vi "Pre Launch Init.vi"(11 "仿真双风扇":refnum<class "Simulated Dual Fan.lvclass">) -> (0 "error out":cluster{"状态":bool, "代码":i32, "源":string} caption="错误输出", 3 "仿真双风扇":refnum<class "Simulated Dual Fan.lvclass">)   [LabVIEW 2015, in "Simulated Dual Fan.lvclass"]
uses:
  Simulated Dual Fan.lvclass
  Cooler Plug-Ins/Simulated Evaporative Cooler.lvclass/Simulation Data_Global.vi
  Dual Fan/Dual Fan/Dual Fan.lvclass
  Cooler Plug-Ins/Simulated Evaporative Cooler.lvclass/Simulated Evaporative Cooler.lvclass
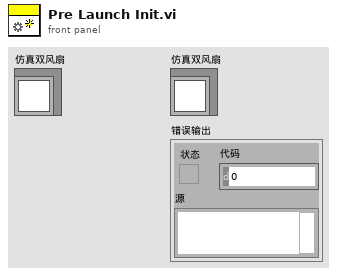
[diagram p1: front panel]
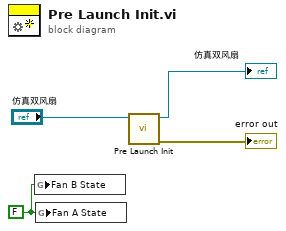
[diagram p0: block diagram]
diagram:
  w2 = FALSE
  n1 = global write "Simulation Data_Global.vi" "Fan B State"(w2) -> ()
  n2 = global write "Simulation Data_Global.vi" "Fan A State"(w2) -> ()
  n3 = call-parent "Pre Launch Init.vi"("定时循环控制器输入"="仿真双风扇") -> ("error out"=→"error out":cluster{"状态":bool, "代码":i32, "源":string}, "定时循环控制器输出"=→"仿真双风扇":refnum<class "Simulated Dual Fan.lvclass">)  [unwired: 9 in]
